vi "send 1 scan poly.vi"   [LabVIEW 2019]
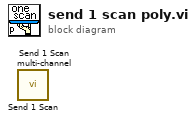
[diagram p0: block diagram]
diagram:
  n1 = call "Send 1 Scan.vi"() -> ()  [unwired: 8 in, 8 out]
  n2 = call "Send 1 Scan multi-channel.vi"() -> ()  [unwired: 8 in, 8 out]
